vi "StartXYPISLoops.vi"(8 "error in (no error)":errorcluster, 9 "Y PIS Controls":T1, 10 "X PIS Controls":T1, 11 "Asylum_Driver in":refnum<class "Asylum_Driver.lvclass">) -> (0 "error out":errorcluster, 3 "Asylum_Driver out":refnum<class "Asylum_Driver.lvclass">)   [LabVIEW 2019, in "Asylum_Driver.lvclass"]
uses:
  Asylum_Driver.lvclass
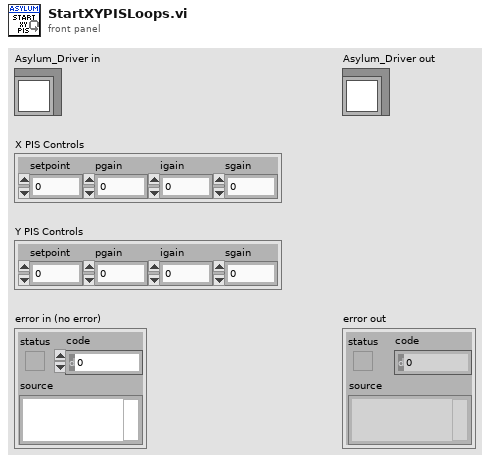
[diagram p1: front panel]
types:
  T1 = cluster{"setpoint":dbl, "pgain":dbl, "igain":dbl, "sgain":dbl}
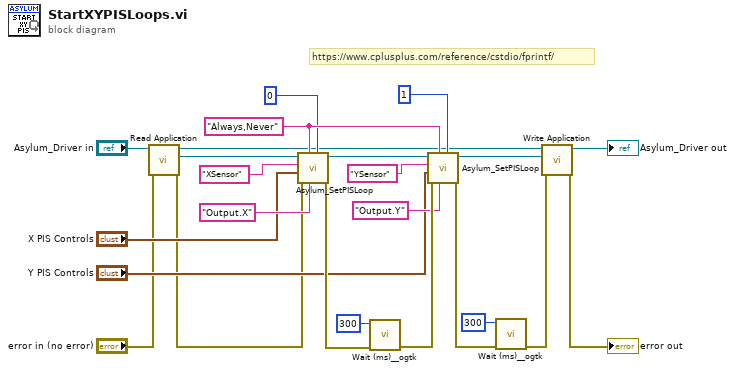
[diagram p0: block diagram]
diagram:
  w22 = "Always,Never" ("eventString")
  # "https://www.cplusplus.com/reference/cstdio/fprintf/"
  n1 = call-dynamic "Read Application.vi"("error in (no error)"="error in (no error)", "Asylum_Driver in"="Asylum_Driver in") -> ("error out"=w3:errorcluster, "Application"=w4:refnum<k7>, "Asylum_Driver out"=w5:refnum<class "Asylum_Driver.lvclass">)  [unwired: 7 in]
  n2 = call <userlib>:"Asylum_SetPISLoop.vi"("whichLoop"=0, "outChannelString"="Output.X", "eventString"=w22, "error in (no error)"=w3, "PIS Controls"="X PIS Controls", "inChannelString"="XSensor", "Application"=w4) -> ("error out"=w23:errorcluster, "Application"=w17:refnum<k7>)  [unwired: 3 in]
  n3 = call <userlib>:"Wait (ms)__ogtk.vi"("error in (no error)"=w23, "milliseconds to wait"=u32 300) -> ("error out"=w24:errorcluster)  [unwired: 8 in, 1 out]
  n4 = call <userlib>:"Asylum_SetPISLoop.vi"("whichLoop"=1, "outChannelString"="Output.Y", "eventString"=w22, "error in (no error)"=w24, "PIS Controls"="Y PIS Controls", "inChannelString"="YSensor", "Application"=w17) -> ("error out"=w12:errorcluster, "Application"=w8:refnum<k7>)  [unwired: 3 in]
  n5 = call <userlib>:"Wait (ms)__ogtk.vi"("error in (no error)"=w12, "milliseconds to wait"=u32 300) -> ("error out"=w7:errorcluster)  [unwired: 8 in, 1 out]
  n6 = call-dynamic "Write Application.vi"("error in (no error)"=w7, "Application"=w8, "Asylum_Driver in"=w5) -> ("error out"=→"error out":errorcluster, "Asylum_Driver out"=→"Asylum_Driver out":refnum<class "Asylum_Driver.lvclass">)  [unwired: 7 in]
